vi "Report Invalid Aliases.vi"(8 "error in (no error)":errorcluster, 10 "Missing Identifiers":T3[](array[typedef]), 11 "Routing and Faulting Custom Device Ref in":T4 format="%.0x") -> (0 "error out":errorcluster, 1 "Aliases Errors":errorcluster[](array[cluster]), 2 "Invalid Aliases":T1[](array[typedef]), 3 "Routing and Faulting Custom Device Ref out":T4 format="%.0x")   [LabVIEW 2017, in "Routing and Faulting Scripting.lvlib"]
uses:
  Routing and Faulting Scripting.lvlib
  <vilib>/NI Veristand/Custom Device API/Custom Device Item Ref.ctl
  Identifier Path Pair.ctl
  Shared/Alias Mapping.ctl
  Shared/Alias Endpoint.ctl
  <vilib>/NI Veristand/Custom Device API/Custom Device API.lvlib
  Shared/Routing and Faulting Shared.lvlib
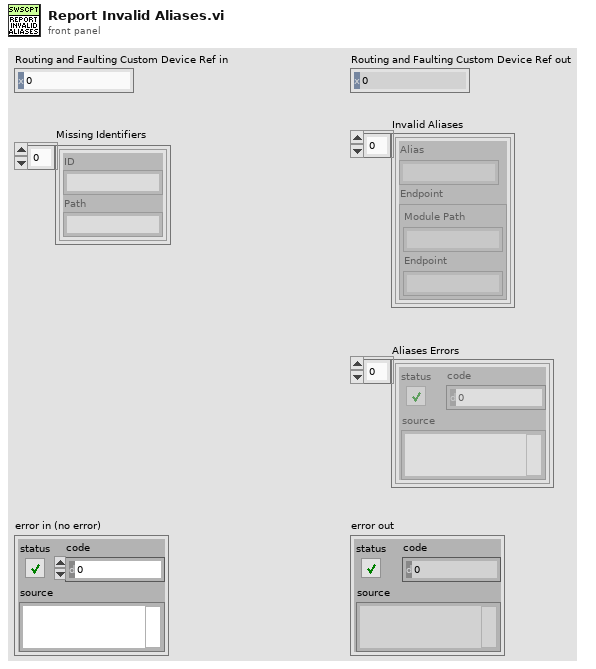
[diagram p1: front panel]
types:
  T1 = typedef "Routing and Faulting Shared.lvlib/Alias Mapping.ctl" = cluster{"Alias":string, "Endpoint":T2}
  T2 = typedef "Routing and Faulting Shared.lvlib/Alias Endpoint.ctl" = cluster{"Module Path":string, "Endpoint":string}
  T3 = typedef "Routing and Faulting Scripting.lvlib/Identifier Path Pair.ctl" = cluster{"ID":string, "Path":string}
  T4 = typedef "Custom Device API.lvlib/Custom Device Item Ref.ctl" = u64
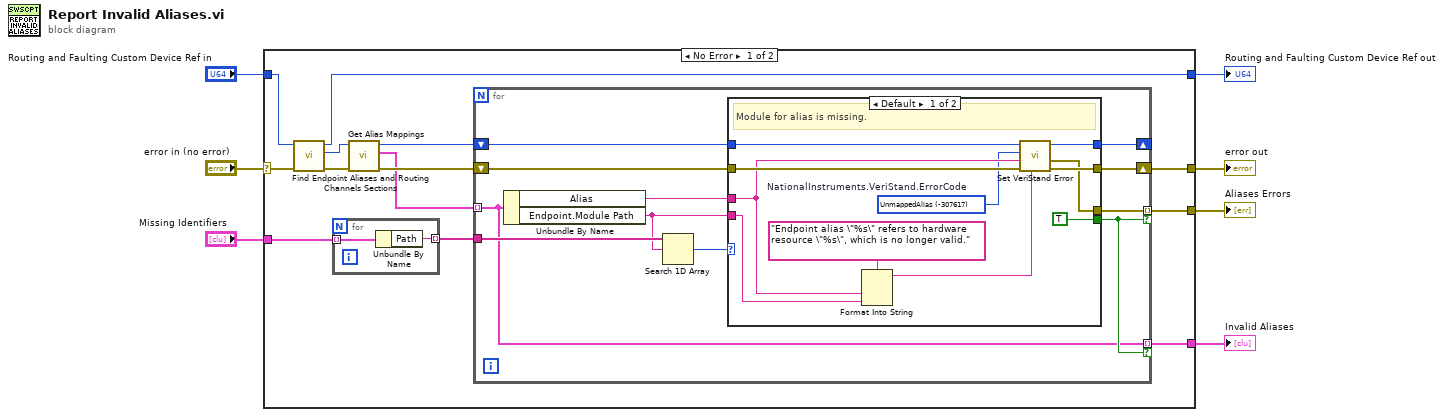
[diagram p0: block diagram]
diagram:
  n1 = case shown="No Error" "error in (no error)" {
    selector: "error in (no error)" -> [w9 w48]
    tunnel: "Routing and Faulting Custom Device Ref in" -> [w15 w47]
    tunnel: [w16 w48] -> w6
    tunnel: [w8 w47] -> w5
    tunnel: "Missing Identifiers" -> [w13 _]
    tunnel: [w11 _] -> w3
    tunnel: [w10 _] -> w2
    frame No Error {
      n2 = call "Find Endpoint Aliases and Routing Channels Sections.vi"("error in (no error)"=w9, "Routing and Faulting Custom Device Ref in"=w15) -> ("error out"=w20:errorcluster, "Endpoint Aliases Ref"=w19:T4, "Routing and Faulting Custom Device Ref out"=w8:T4)  [unwired: 6 in, 1 out]
      n3 = for {
        tunnel: w13 -> [w22] mode=indexing
        tunnel: [w21] -> w12 mode=indexing
        n4 = Unbundle By Name(w22) -> ("Path"=w21:string)
      }
      n5 = call "Get Alias Mappings.vi"("error in (no error)"=w20, "Endpoint Aliases Ref in"=w19) -> ("error out"=w18:errorcluster, "Alias Mappings"=w14:T1[], "Endpoint Aliases Ref out"=w17:T4)  [unwired: 7 in]
      n6 = for {
        tunnel: w14 -> [w25] mode=indexing
        tunnel: w12 -> [w33]
        tunnel: [w25] -> w10 mode=indexing if=w26
        shift-right: [w30] -> w16
        shift-left: w18 -> [w31]
        tunnel: [w27] -> w11 mode=indexing if=w26
        shift-right: [w23] -> _
        shift-left: w17 -> [w24]
        n7 = Unbundle By Name(w25) -> ("Alias"=w29:string, "Endpoint.Module Path"=w28:string)
        n8 = Search 1D Array(1D array=w33, element=w28) -> (index of element=w32:i32)  [unwired: 1 in]
        n9 = case shown="Default" w32 {
          tunnel: w29 -> [w42 _]
          tunnel: w31 -> [w44 w46]
          tunnel: [w43 w46] -> w30
          tunnel: [TRUE _] -> w26
          tunnel: w28 -> [w41 _]
          tunnel: [w39 _] -> w27
          tunnel: w24 -> [w38 w45]
          tunnel: [w34 w45] -> w23
          frame Default {
            w37 = -307617 items=["Success"=0, "NoProjectOpen"=-307992, "SequenceCompileError"=-307988, "SessionAlreadyDeployed"=-307984, "SessionNotDeployed"=-307982, "SequenceNotFoundInSession"=-307981, "StimulusProfileSessionLocked"=-307980, "EmptyNodeName"=-307930, "NodeAlreadyExistsByName"=-307926, "NumberOfCoefficientsOutOfRange"=-307884, "DownloadFileError"=-307872, "IncorrectLogFileName"=-307871, "LogTriggerConditionSyntaxError"=-307868, "DuplicateLogSessionName"=-307867, "LogSessionNotFound"=-307865, "ChannelLengthMismatch"=-307830, "NodeNotFoundDuringCompile"=-307829, "ChannelNodeRemoved"=-307828, "NotAChannel"=-307825, "NotAWaveform"=-307824, "STIFileError"=-307784, "DependenciesCycle"=-307783, "ChannelNotFoundInLogFile"=-307782, "ChannelGroupNotFoundInLogFile"=-307781, "GatewayNotOnLocalhost"=-307780, "NotEnoughDynamicDataSharingSpace"=-307738, "TargetMissingDataSharingDevice"=-307737, "ChannelMappingsSizeMismatch"=-307728, "DuplicateChannelAliasMappings"=-307711, "NotAnInlineCustomDevice"=-307710, "IncompatibleModel"=-307703, "ModelDimensionMismatch"=-307702, "SLSCChassisLoadFailed"=-307691, "TargetDisabled"=-307689, "MismatchedLengths"=-307687, "TargetInvalid"=-307686, "ParameterNotFound"=-307685, "ServerPortAlreadyInUse"=-307684, "TargetDisconnected"=-307682, "ServiceConfigurationFile"=-307681, "ModelParameterFileParseError"=-307680, "NoActionRequired"=-307677, "InputParameterInvalid"=-307676, "HostRunningDifferentSystemDefinition"=-307671, "ChannelNotScalable"=-307668, "ChannelCannotBeFaulted"=-307666, "ChannelNotWritable"=-307665, "ChannelNotReadable"=-307664, "Timeout"=-307663, "NodeNotFound"=-307662, "SystemDefinitionDeploymentFailure"=-307661, "SystemDefinitionDeploymentTimeout"=-307660, "EmptyPassword"=-307659, "SystemDefinitionAlreadyActive"=-307658, "InvalidConfigurationPassword"=-307657, "NoSystemDefinitionLoaded"=-307656, "ComponentNotAvailable"=-307655, "NotDeployed"=-307654, "InvalidFile"=-307653, "FailedServerConnection"=-307652, "FunctionNotSupported"=-307651, "UnexpectedError"=-307650, "UnmappedAlias"=-307617, "InvalidStreamConditionForDataType"=-307554, "WaveformDataTypeMismatch"=-307553, "InvalidDaqPluginFile"=-307526, "FileVersionUnsupported"=-307525]  # NationalInstruments.VeriStand.ErrorCode
            # "Module for alias is missing."
            n10 = Format Into String(format string="Endpoint alias \"%s\" refers to hardware resource \"%s\", which is no longer valid.", w42, w41) -> (resulting string=w35:string)  [unwired: 2 in, 1 out]
            n11 = call "Set VeriStand Error.vi"("message"=w35, "error in (no error)"=w44, "key"=w42, "errCode"=w37, "Custom Device Item Ref in"=w38) -> ("error out"=w43:errorcluster, "VeriStand Error out"=w39:errorcluster, "Custom Device Item Ref out"=w34:T4)  [unwired: 4 in]
          }
          frame -1 {
            # "Module still exists. Validate endpoint."
          }
        }
      }
    }
    frame Error {
    }
  }
  "Routing and Faulting Custom Device Ref out" <- w5
  "error out" <- w6
  "Aliases Errors" <- w3
  "Invalid Aliases" <- w2
